vi "Set Oven Temperature.vi"(8 "error in":errorcluster, 10 "Oven Temperature":i32, 11 "OVG In":refnum<class "Owlstone GEN-SYS.lvclass">) -> (0 "error out":errorcluster, 3 "OVG Out":refnum<class "Owlstone GEN-SYS.lvclass">)   [LabVIEW 2011, in "Owlstone GEN-SYS.lvclass"]
uses:
  Owlstone GEN-SYS.lvclass
  Owlstone GEN-SYS.lvclass/Owlstone GEN-SYS.ctl
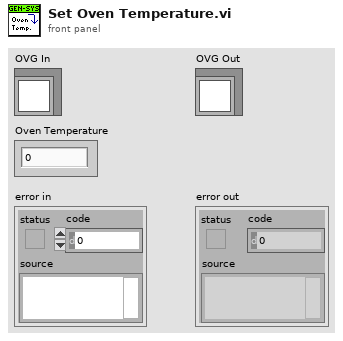
[diagram p1: front panel]
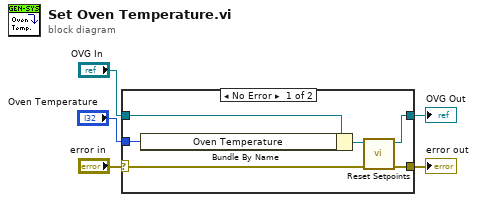
[diagram p0: block diagram]
diagram:
  n1 = case shown="No Error" "error in" {
    selector: "error in" -> [w7 w13]
    tunnel: "Oven Temperature" -> [w10 _]
    tunnel: [w6 w13] -> w3
    tunnel: "OVG In" -> [w11 w12]
    tunnel: [w8 w12] -> w1
    frame No Error {
      n2 = Bundle By Name(cluster=w11, "Oven Temperature"=w10) -> (w9:refnum<class "Owlstone GEN-SYS.lvclass">)
      n3 = call "Reset Setpoints.vi"("error in (no error)"=w7, "Owlstone GEN-SYS in"=w9) -> ("error out"=w6:errorcluster, "Owlstone GEN-SYS out"=w8:refnum<class "Owlstone GEN-SYS.lvclass">)  [unwired: 8 in]
    }
    frame Error {
    }
  }
  "error out" <- w3
  "OVG Out" <- w1
